vi "Binary Bad Tube Search SubVI.vi"() -> ()   [LabVIEW 2020]
panel:
  in  "Number of Active tubes":i32
  out "Sync Pin Task Out":refnum<k21>
  out "Write Pin Task Out":refnum<k21>
  out "Data Pin Task Out":refnum<k21>
  out "Clear Pin Task Out":refnum<k21>
  in  "Clear Pin Task In":refnum<k21>
  in  "Data Pin Task In":refnum<k21>
  in  "Sync Pin Task In":refnum<k21>
  in  "Write Pin Task In":refnum<k21>
  in  "Dark Current (all tubes)":dbl
  # "Necessary"
  # "Necessary"
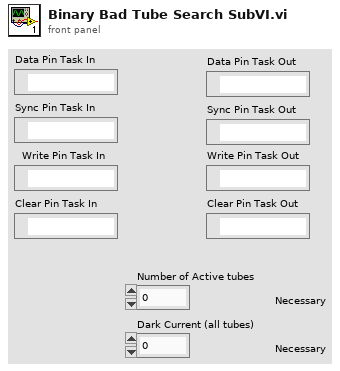
[diagram p1: front panel]
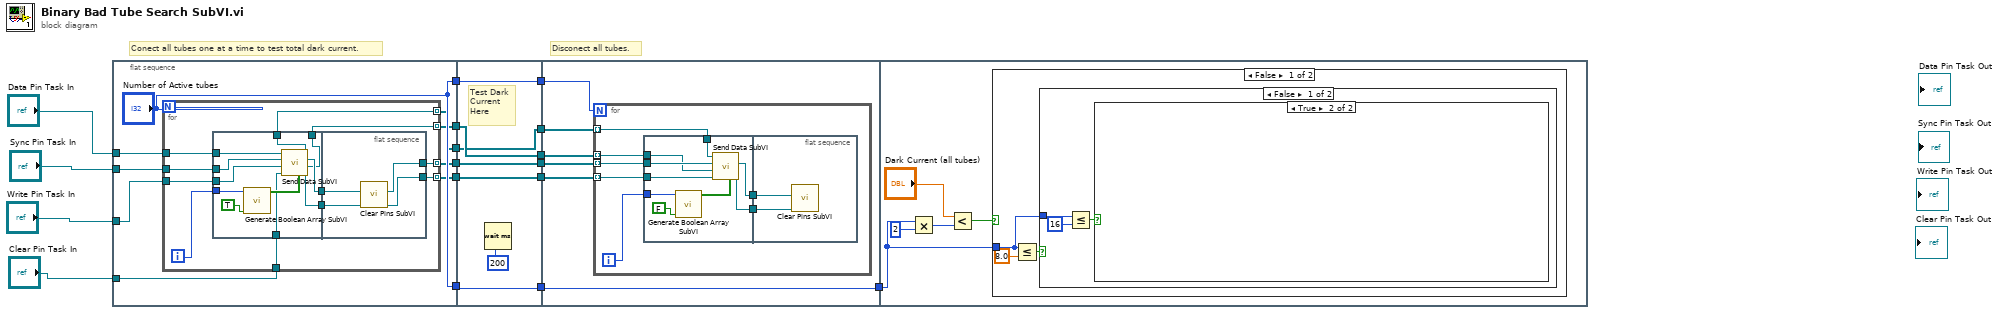
[diagram p0: block diagram]
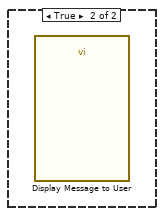
[diagram p4: hidden frame]
diagram:
  # "Disconect all tubes."
  # "Conect all tubes one at a time to test total dark current."
  n1 = flat-sequence {
    tunnel: "Data Pin Task In" -> [w26]
    tunnel: "Sync Pin Task In" -> [w25]
    tunnel: "Write Pin Task In" -> [w24]
    tunnel: "Clear Pin Task In" -> [w23]
    tunnel: ["Number of Active tubes"] -> w13
    tunnel: ["Number of Active tubes"] -> w9
    tunnel: [w21] -> w7
    tunnel: [w20] -> w5
    tunnel: [w19] -> w3
    tunnel: [w18] -> w1
    tunnel: w13 -> [w59]
    tunnel: [w59] -> w12
    tunnel: [w57] -> w10
    tunnel: w9 -> [w57]
    tunnel: [w56] -> w8
    tunnel: w7 -> [w56]
    tunnel: [w55] -> w6
    tunnel: w5 -> [w55]
    tunnel: [w54] -> w4
    tunnel: w3 -> [w54]
    tunnel: [w53] -> w2
    tunnel: w1 -> [w53]
    tunnel: w12 -> [w65]
    tunnel: [w65] -> w11
    tunnel: w10 -> [w64]
    tunnel: w8 -> [w63]
    tunnel: w6 -> [w62]
    tunnel: w4 -> [w61]
    tunnel: w2 -> [w60]
    tunnel: w11 -> [w84]
    frame #0 {
      n2 = for {
        N: "Number of Active tubes" -> [_]
        tunnel: w26 -> [w36]
        tunnel: w25 -> [w35]
        tunnel: w24 -> [w34]
        tunnel: w23 -> [w33]
        tunnel: [w30] -> w21 mode=indexing
        tunnel: [w29] -> w20 mode=indexing
        tunnel: [w28] -> w19 mode=indexing
        tunnel: [w27] -> w18 mode=indexing
        i -> [w37]
        n3 = flat-sequence {
          tunnel: w37 -> [w46]
          tunnel: w36 -> [w45]
          tunnel: w35 -> [w44]
          tunnel: w34 -> [w43]
          tunnel: w33 -> [w42]
          tunnel: [w41] -> w32
          tunnel: [w40] -> w31
          tunnel: [w39] -> w28
          tunnel: [w38] -> w27
          tunnel: w32 -> [w52]
          tunnel: w31 -> [w51]
          tunnel: [w50] -> w30
          tunnel: [w49] -> w29
          frame #0 {
            n4 = call "Generate Boolean Array SubVI.vi"("Activate: 1\nDeactivate: 0"=TRUE, "Tube"=w46) -> ("Boolean array"=w47:bool[])  [unwired: 9 in]
            n5 = call "Send Data SubVI.vi"("Data Pin Task In"=w45, "Sync Pin Task In"=w44, "Write Pin Task In"=w43, "Clear Pin Task In"=w42, "Data"=w47) -> ("Data Pin Task Out"=w38:refnum<k21>, "Sync Pin Task Out"=w41:refnum<k21>, "Write Pin Task Out"=w39:refnum<k21>, "Clear Pin Task Out"=w40:refnum<k21>)  [unwired: 1 in]
          }
          frame #1 {
            n6 = call "Clear Pins SubVI.vi"("Clear Pin Task In"=w51, "Sync Pin Task In"=w52) -> ("Clear Pin Task Out"=w49:refnum<k21>, "Sync Pin Task Out"=w50:refnum<k21>)  [unwired: 8 in]
          }
        }
      }
    }
    frame #1 {
      # "Test Dark \nCurrent \nHere"
      n7 = Wait (ms)(milliseconds to wait=u32 200) -> ()  [unwired: 1 out]
    }
    frame #2 {
      n8 = for {
        N: w64 -> [_]
        tunnel: w63 -> [w69] mode=indexing
        tunnel: w62 -> [w68] mode=indexing
        tunnel: w61 -> [w67] mode=indexing
        tunnel: w60 -> [w66] mode=indexing
        i -> [w72]
        n9 = flat-sequence {
          tunnel: w72 -> [w79]
          tunnel: [w78] -> w71
          tunnel: [w77] -> w70
          tunnel: w69 -> [w76]
          tunnel: w68 -> [w75]
          tunnel: w67 -> [w74]
          tunnel: w66 -> [w73]
          tunnel: w71 -> [w83]
          tunnel: w70 -> [w82]
          frame #0 {
            n10 = call "Generate Boolean Array SubVI.vi"("Activate: 1\nDeactivate: 0"=FALSE, "Tube"=w79) -> ("Boolean array"=w80:bool[])  [unwired: 9 in]
            n11 = call "Send Data SubVI.vi"("Data Pin Task In"=w73, "Sync Pin Task In"=w76, "Write Pin Task In"=w74, "Clear Pin Task In"=w75, "Data"=w80) -> ("Sync Pin Task Out"=w78:refnum<k21>, "Clear Pin Task Out"=w77:refnum<k21>)  [unwired: 1 in, 2 out]
          }
          frame #1 {
            n12 = call "Clear Pins SubVI.vi"("Clear Pin Task In"=w82, "Sync Pin Task In"=w83) -> ()  [unwired: 8 in, 2 out]
          }
        }
      }
    }
    frame #3 {
      n13 = Multiply(x=w84, y=2) -> (x*y=w85:i32)
      n14 = Less?(x="Dark Current (all tubes)", y=w85) -> (x < y?=w87:bool)
      n15 = case shown="False" w87 {
        tunnel: w84 -> [w89 _]
        frame False {
          n16 = Less Or Equal?(x=w89, y=8.0) -> (x <= y?=w90:bool)
          n17 = case shown="False" w90 {
            tunnel: w89 -> [w94 _]
            frame False {
              n18 = Less Or Equal?(x=w94, y=16) -> (x <= y?=w92:bool)
              n19 = case shown="True" w92 {
                frame False {
                }
                frame True {
                }
              }
            }
            frame True {
            }
          }
        }
        frame True {
          n20 = call "Display Message to User"() -> ()  [unwired: 10 in, 2 out]
        }
      }
    }
  }
